vi "Sort 2D String Array - Sort Data.vi"(0 "Array to sort in":string[][](array[string]), 3 "Column Sort Order":i32[](array[numeric]), 4 "Input Array Contains Header Row? (T)":T1) -> (14 "Sorted Array (Cols in Original Order. Header row removed)":T2, 15 "Sorted Array (Cols in Sort Order. Header row removed)":T4, 16 "Sorted Array (Cols in Sort Order. Headers as last row)":T3)   [LabVIEW 2009, in "xijk_select_best_filter.lvlib"]
doc: "Sort 2D String Array - Sort Data.vi\n\n<B>Description:</B>\n\nThis VI sorts an array of strings in the order specified by the Column Sort Order input.\n\n<B>Usage:</B>\n\nWire all required inputs.\n\n<B>Inputs:</B>\n\nArray to Sort In\n- This is the input array of strings that will be sorted.\n\nColumn Sort Order\n- This control specifies the column sort order. If it is left unwired, the sort order will be 0,1,2...\n\nInput Array Contains Header Row? (T)\n- This input indicates if the input array contains a header row.\n\n<B>Outputs:</B>\n\nSorted Array (Cols in Original Order. Header row removed)\n- This is the input array of strings sorted in the order specified by the Column Sort Order input with the columns in the original order and the header row removed.\n\nSorted Array (Cols in Sort Order. Header row removed)\n- This is the input array of strings sorted in the order specified by the Column Sort Order input with the columns in the order specified by the Column Sort Order input and the header row removed.\n\nSorted Array (Cols in Sort Order. Headers as last row)\n- This is the input array of strings sorted in the order specified by the Column Sort Order input with the columns in the order specified by the Column Sort Order input and the header row positioned as the last row of the array.\n\n<B>Developed by:</B>\n\nMark Ridgley\nmark.ridgley@logicpd.com"
uses:
  xijk_select_best_filter.lvlib
  _TypeDefs/TYPE - Sorted Array (Cols in Original Order. Header row removed).ctl
  _TypeDefs/TYPE - Sorted Array (Cols in Sort Order. Header row removed).ctl
  _TypeDefs/TYPE - Sorted Array (Cols in Sort Order. Headers as last row).ctl
  _TypeDefs/TYPE - Input Array Contains Header Row.ctl
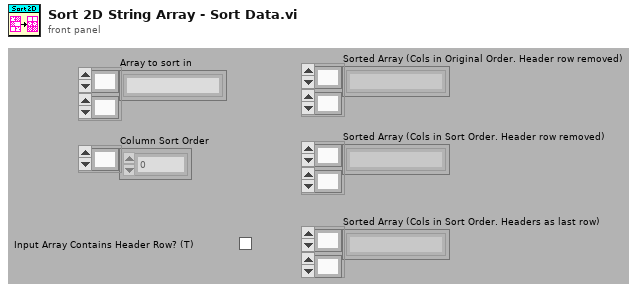
[diagram p1: front panel]
types:
  T1 = typedef "xijk_select_best_filter.lvlib/TYPE - Input Array Contains Header Row.ctl" = bool
  T2 = typedef "xijk_select_best_filter.lvlib/TYPE - Sorted Array (Cols in Original Order. Header row removed).ctl" = string[][]
  T3 = typedef "xijk_select_best_filter.lvlib/TYPE - Sorted Array (Cols in Sort Order. Headers as last row).ctl" = string[][]
  T4 = typedef "xijk_select_best_filter.lvlib/TYPE - Sorted Array (Cols in Sort Order. Header row removed).ctl" = string[][]
  T5 = cluster{"Output String (\" \")":string, "Output String (\" \")":string, "Output String (\" \")":string, "Output String (\" \")":string, "Output String (\" \")":string, "Output String (\" \")":string, "Output String (\" \")":string, "Output String (\" \")":string, "Output String (\" \")":string, "Output String (\" \")":string, "Output String (\" \")":string, "Output String (\" \")":string, "Output String (\" \")":string, "Output String (\" \")":string, "Output String (\" \")":string, "Output String (\" \")":string, "Output String (\" \")":string, "Output String (\" \")":string, "Output String (\" \")":string, "Output String (\" \")":string, "Output String (\" \")":string, "Output String (\" \")":string, "Output String (\" \")":string, "Output String (\" \")":string, "Output String (\" \")":string, "Output String (\" \")":string, "Output String (\" \")":string, "Output String (\" \")":string, "Output String (\" \")":string, "Output String (\" \")":string, "Output String (\" \")":string, "Output String (\" \")":string, "Output String (\" \")":string, "Output String (\" \")":string, "Output String (\" \")":string, "Output String (\" \")":string, "Output String (\" \")":string, "Output String (\" \")":string, "Output String (\" \")":string, "Output String (\" \")":string, "Output String (\" \")":string, "Output String (\" \")":string, "Output String (\" \")":string, "Output String (\" \")":string, "Output String (\" \")":string, "Output String (\" \")":string, "Output String (\" \")":string, "Output String (\" \")":string, "Output String (\" \")":string, "Output String (\" \")":string, "Output String (\" \")":string, "Output String (\" \")":string, "Output String (\" \")":string, "Output String (\" \")":string, "Output String (\" \")":string, "Output String (\" \")":string, "Output String (\" \")":string, "Output String (\" \")":string, "Output String (\" \")":string, "Output String (\" \")":string, "Output String (\" \")":string, "Output String (\" \")":string, "Output String (\" \")":string, "Output String (\" \")":string, "Output String (\" \")":string, "Output String (\" \")":string, "Output String (\" \")":string, "Output String (\" \")":string, "Output String (\" \")":string, "Output String (\" \")":string, "Output String (\" \")":string, "Output String (\" \")":string, "Output String (\" \")":string, "Output String (\" \")":string, "Output String (\" \")":string, "Output String (\" \")":string, "Output String (\" \")":string, "Output String (\" \")":string, "Output String (\" \")":string, "Output String (\" \")":string, "Output String (\" \")":string, "Output String (\" \")":string, "Output String (\" \")":string, "Output String (\" \")":string, "Output String (\" \")":string, "Output String (\" \")":string, "Output String (\" \")":string, "Output String (\" \")":string, "Output String (\" \")":string, "Output String (\" \")":string, "Output String (\" \")":string, "Output String (\" \")":string, "Output String (\" \")":string, "Output String (\" \")":string, "Output String (\" \")":string, "Output String (\" \")":string, "Output String (\" \")":string, "Output String (\" \")":string, "Output String (\" \")":string, "Output String (\" \")":string, "Output String (\" \")":string, "Output String (\" \")":string, "Output String (\" \")":string, "Output String (\" \")":string, "Output String (\" \")":string, "Output String (\" \")":string, "Output String (\" \")":string, "Output String (\" \")":string, "Output String (\" \")":string, "Output String (\" \")":string, "Output String (\" \")":string, "Output String (\" \")":string, "Output String (\" \")":string, "Output String (\" \")":string, "Output String (\" \")":string, "Output String (\" \")":string, "Output String (\" \")":string, "Output String (\" \")":string, "Output String (\" \")":string, "Output String (\" \")":string, "Output String (\" \")":string, "Output String (\" \")":string, "Output String (\" \")":string, "Output String (\" \")":string, "Output String (\" \")":string, "Output String (\" \")":string, "Output String (\" \")":string, "Output String (\" \")":string, "Output String (\" \")":string, "Output String (\" \")":string, "Output String (\" \")":string, "Output String (\" \")":string, "Output String (\" \")":string, "Output String (\" \")":string, "Output String (\" \")":string, "Output String (\" \")":string, "Output String (\" \")":string, "Output String (\" \")":string, "Output String (\" \")":string, "Output String (\" \")":string, "Output String (\" \")":string, "Output String (\" \")":string, "Output String (\" \")":string, "Output String (\" \")":string, "Output String (\" \")":string, "Output String (\" \")":string, "Output String (\" \")":string, "Output String (\" \")":string, "Output String (\" \")":string, "Output String (\" \")":string, "Output String (\" \")":string, "Output String (\" \")":string, "Output String (\" \")":string, "Output String (\" \")":string, "Output String (\" \")":string, "Output String (\" \")":string, "Output String (\" \")":string, "Output String (\" \")":string, "Output String (\" \")":string, "Output String (\" \")":string, "Output String (\" \")":string, "Output String (\" \")":string, "Output String (\" \")":string, "Output String (\" \")":string, "Output String (\" \")":string, "Output String (\" \")":string, "Output String (\" \")":string, "Output String (\" \")":string, "Output String (\" \")":string, "Output String (\" \")":string, "Output String (\" \")":string, "Output String (\" \")":string, "Output String (\" \")":string, "Output String (\" \")":string, "Output String (\" \")":string, "Output String (\" \")":string, "Output String (\" \")":string, "Output String (\" \")":string, "Output String (\" \")":string, "Output String (\" \")":string, "Output String (\" \")":string, "Output String (\" \")":string, "Output String (\" \")":string, "Output String (\" \")":string, "Output String (\" \")":string, "Output String (\" \")":string, "Output String (\" \")":string, "Output String (\" \")":string, "Output String (\" \")":string, "Output String (\" \")":string, "Output String (\" \")":string, "Output String (\" \")":string, "Output String (\" \")":string, "Output String (\" \")":string, "Output String (\" \")":string, "Output String (\" \")":string, "Output String (\" \")":string, "Output String (\" \")":string, "Output String (\" \")":string, "Output String (\" \")":string, "Output String (\" \")":string, "Output String (\" \")":string, "Output String (\" \")":string, "Output String (\" \")":string, "Output String (\" \")":string, "Output String (\" \")":string, "Output String (\" \")":string, "Output String (\" \")":string, "Output String (\" \")":string, "Output String (\" \")":string, "Output String (\" \")":string, "Output String (\" \")":string, "Output String (\" \")":string, "Output String (\" \")":string, "Output String (\" \")":string, "Output String (\" \")":string, "Output String (\" \")":string, "Output String (\" \")":string, "Output String (\" \")":string, "Output String (\" \")":string, "Output String (\" \")":string, "Output String (\" \")":string, "Output String (\" \")":string, "Output String (\" \")":string, "Output String (\" \")":string, "Output String (\" \")":string, "Output String (\" \")":string, "Output String (\" \")":string, "Output String (\" \")":string, "Output String (\" \")":string, "Output String (\" \")":string, "Output String (\" \")":string, "Output String (\" \")":string, "Output String (\" \")":string, "Output String (\" \")":string, "Output String (\" \")":string, "Output String (\" \")":string, "Output String (\" \")":string, "Output String (\" \")":string, "Output String (\" \")":string, "Output String (\" \")":string, "Output String (\" \")":string, "Output String (\" \")":string, "Output String (\" \")":string, "Output String (\" \")":string, "Output String (\" \")":string, "Output String (\" \")":string, "Output String (\" \")":string, "Output String (\" \")":string, "Output String (\" \")":string, "Output String (\" \")":string, "Output String (\" \")":string, "Output String (\" \")":string, "Output String (\" \")":string, "Output String (\" \")":string, "Output String (\" \")":string}[]
  T6 = cluster{"[0]":string, "[1]":string, "[2]":string, "[3]":string, "[4]":string, "[5]":string, "[6]":string, "[7]":string, "[8]":string, "[9]":string, "[10]":string, "[11]":string, "[12]":string, "[13]":string, "[14]":string, "[15]":string, "[16]":string, "[17]":string, "[18]":string, "[19]":string, "[20]":string, "[21]":string, "[22]":string, "[23]":string, "[24]":string, "[25]":string, "[26]":string, "[27]":string, "[28]":string, "[29]":string, "[30]":string, "[31]":string, "[32]":string, "[33]":string, "[34]":string, "[35]":string, "[36]":string, "[37]":string, "[38]":string, "[39]":string, "[40]":string, "[41]":string, "[42]":string, "[43]":string, "[44]":string, "[45]":string, "[46]":string, "[47]":string, "[48]":string, "[49]":string, "[50]":string, "[51]":string, "[52]":string, "[53]":string, "[54]":string, "[55]":string, "[56]":string, "[57]":string, "[58]":string, "[59]":string, "[60]":string, "[61]":string, "[62]":string, "[63]":string, "[64]":string, "[65]":string, "[66]":string, "[67]":string, "[68]":string, "[69]":string, "[70]":string, "[71]":string, "[72]":string, "[73]":string, "[74]":string, "[75]":string, "[76]":string, "[77]":string, "[78]":string, "[79]":string, "[80]":string, "[81]":string, "[82]":string, "[83]":string, "[84]":string, "[85]":string, "[86]":string, "[87]":string, "[88]":string, "[89]":string, "[90]":string, "[91]":string, "[92]":string, "[93]":string, "[94]":string, "[95]":string, "[96]":string, "[97]":string, "[98]":string, "[99]":string, "[100]":string, "[101]":string, "[102]":string, "[103]":string, "[104]":string, "[105]":string, "[106]":string, "[107]":string, "[108]":string, "[109]":string, "[110]":string, "[111]":string, "[112]":string, "[113]":string, "[114]":string, "[115]":string, "[116]":string, "[117]":string, "[118]":string, "[119]":string, "[120]":string, "[121]":string, "[122]":string, "[123]":string, "[124]":string, "[125]":string, "[126]":string, "[127]":string, "[128]":string, "[129]":string, "[130]":string, "[131]":string, "[132]":string, "[133]":string, "[134]":string, "[135]":string, "[136]":string, "[137]":string, "[138]":string, "[139]":string, "[140]":string, "[141]":string, "[142]":string, "[143]":string, "[144]":string, "[145]":string, "[146]":string, "[147]":string, "[148]":string, "[149]":string, "[150]":string, "[151]":string, "[152]":string, "[153]":string, "[154]":string, "[155]":string, "[156]":string, "[157]":string, "[158]":string, "[159]":string, "[160]":string, "[161]":string, "[162]":string, "[163]":string, "[164]":string, "[165]":string, "[166]":string, "[167]":string, "[168]":string, "[169]":string, "[170]":string, "[171]":string, "[172]":string, "[173]":string, "[174]":string, "[175]":string, "[176]":string, "[177]":string, "[178]":string, "[179]":string, "[180]":string, "[181]":string, "[182]":string, "[183]":string, "[184]":string, "[185]":string, "[186]":string, "[187]":string, "[188]":string, "[189]":string, "[190]":string, "[191]":string, "[192]":string, "[193]":string, "[194]":string, "[195]":string, "[196]":string, "[197]":string, "[198]":string, "[199]":string, "[200]":string, "[201]":string, "[202]":string, "[203]":string, "[204]":string, "[205]":string, "[206]":string, "[207]":string, "[208]":string, "[209]":string, "[210]":string, "[211]":string, "[212]":string, "[213]":string, "[214]":string, "[215]":string, "[216]":string, "[217]":string, "[218]":string, "[219]":string, "[220]":string, "[221]":string, "[222]":string, "[223]":string, "[224]":string, "[225]":string, "[226]":string, "[227]":string, "[228]":string, "[229]":string, "[230]":string, "[231]":string, "[232]":string, "[233]":string, "[234]":string, "[235]":string, "[236]":string, "[237]":string, "[238]":string, "[239]":string, "[240]":string, "[241]":string, "[242]":string, "[243]":string, "[244]":string, "[245]":string, "[246]":string, "[247]":string, "[248]":string, "[249]":string, "[250]":string, "[251]":string, "[252]":string, "[253]":string, "[254]":string, "[255]":string}
  T7 = cluster{"[0]":string, "[1]":string, "[2]":string, "[3]":string, "[4]":string, "[5]":string, "[6]":string, "[7]":string, "[8]":string, "[9]":string, "[10]":string, "[11]":string, "[12]":string, "[13]":string, "[14]":string, "[15]":string, "[16]":string, "[17]":string, "[18]":string, "[19]":string, "[20]":string, "[21]":string, "[22]":string, "[23]":string, "[24]":string, "[25]":string, "[26]":string, "[27]":string, "[28]":string, "[29]":string, "[30]":string, "[31]":string, "[32]":string, "[33]":string, "[34]":string, "[35]":string, "[36]":string, "[37]":string, "[38]":string, "[39]":string, "[40]":string, "[41]":string, "[42]":string, "[43]":string, "[44]":string, "[45]":string, "[46]":string, "[47]":string, "[48]":string, "[49]":string, "[50]":string, "[51]":string, "[52]":string, "[53]":string, "[54]":string, "[55]":string, "[56]":string, "[57]":string, "[58]":string, "[59]":string, "[60]":string, "[61]":string, "[62]":string, "[63]":string, "[64]":string, "[65]":string, "[66]":string, "[67]":string, "[68]":string, "[69]":string, "[70]":string, "[71]":string, "[72]":string, "[73]":string, "[74]":string, "[75]":string, "[76]":string, "[77]":string, "[78]":string, "[79]":string, "[80]":string, "[81]":string, "[82]":string, "[83]":string, "[84]":string, "[85]":string, "[86]":string, "[87]":string, "[88]":string, "[89]":string, "[90]":string, "[91]":string, "[92]":string, "[93]":string, "[94]":string, "[95]":string, "[96]":string, "[97]":string, "[98]":string, "[99]":string, "[100]":string, "[101]":string, "[102]":string, "[103]":string, "[104]":string, "[105]":string, "[106]":string, "[107]":string, "[108]":string, "[109]":string, "[110]":string, "[111]":string, "[112]":string, "[113]":string, "[114]":string, "[115]":string, "[116]":string, "[117]":string, "[118]":string, "[119]":string, "[120]":string, "[121]":string, "[122]":string, "[123]":string, "[124]":string, "[125]":string, "[126]":string, "[127]":string, "[128]":string, "[129]":string, "[130]":string, "[131]":string, "[132]":string, "[133]":string, "[134]":string, "[135]":string, "[136]":string, "[137]":string, "[138]":string, "[139]":string, "[140]":string, "[141]":string, "[142]":string, "[143]":string, "[144]":string, "[145]":string, "[146]":string, "[147]":string, "[148]":string, "[149]":string, "[150]":string, "[151]":string, "[152]":string, "[153]":string, "[154]":string, "[155]":string, "[156]":string, "[157]":string, "[158]":string, "[159]":string, "[160]":string, "[161]":string, "[162]":string, "[163]":string, "[164]":string, "[165]":string, "[166]":string, "[167]":string, "[168]":string, "[169]":string, "[170]":string, "[171]":string, "[172]":string, "[173]":string, "[174]":string, "[175]":string, "[176]":string, "[177]":string, "[178]":string, "[179]":string, "[180]":string, "[181]":string, "[182]":string, "[183]":string, "[184]":string, "[185]":string, "[186]":string, "[187]":string, "[188]":string, "[189]":string, "[190]":string, "[191]":string, "[192]":string, "[193]":string, "[194]":string, "[195]":string, "[196]":string, "[197]":string, "[198]":string, "[199]":string, "[200]":string, "[201]":string, "[202]":string, "[203]":string, "[204]":string, "[205]":string, "[206]":string, "[207]":string, "[208]":string, "[209]":string, "[210]":string, "[211]":string, "[212]":string, "[213]":string, "[214]":string, "[215]":string, "[216]":string, "[217]":string, "[218]":string, "[219]":string, "[220]":string, "[221]":string, "[222]":string, "[223]":string, "[224]":string, "[225]":string, "[226]":string, "[227]":string, "[228]":string, "[229]":string, "[230]":string, "[231]":string, "[232]":string, "[233]":string, "[234]":string, "[235]":string, "[236]":string, "[237]":string, "[238]":string, "[239]":string, "[240]":string, "[241]":string, "[242]":string, "[243]":string, "[244]":string, "[245]":string, "[246]":string, "[247]":string, "[248]":string, "[249]":string, "[250]":string, "[251]":string, "[252]":string, "[253]":string, "[254]":string, "[255]":string}[]
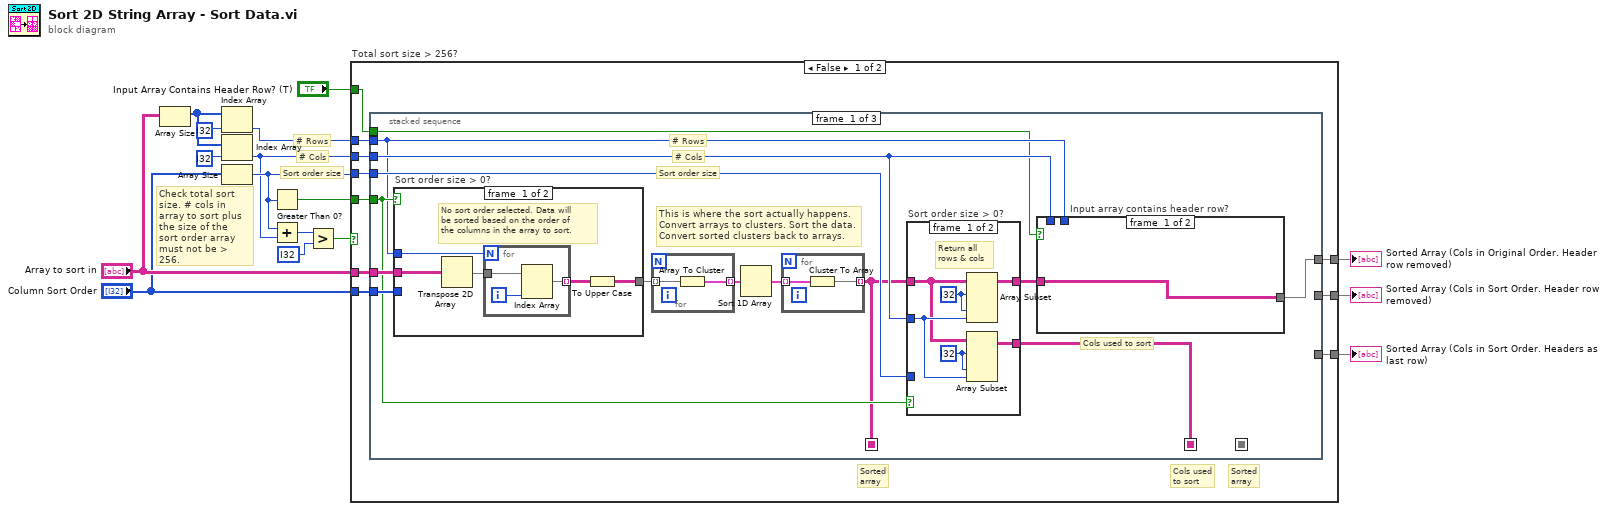
[diagram p0: block diagram]
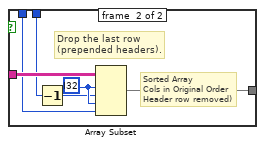
[diagram p2: hidden frame]
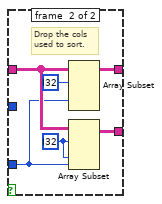
[diagram p3: hidden frame]
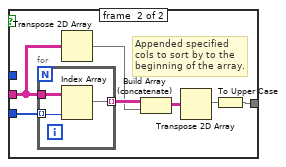
[diagram p4: hidden frame]
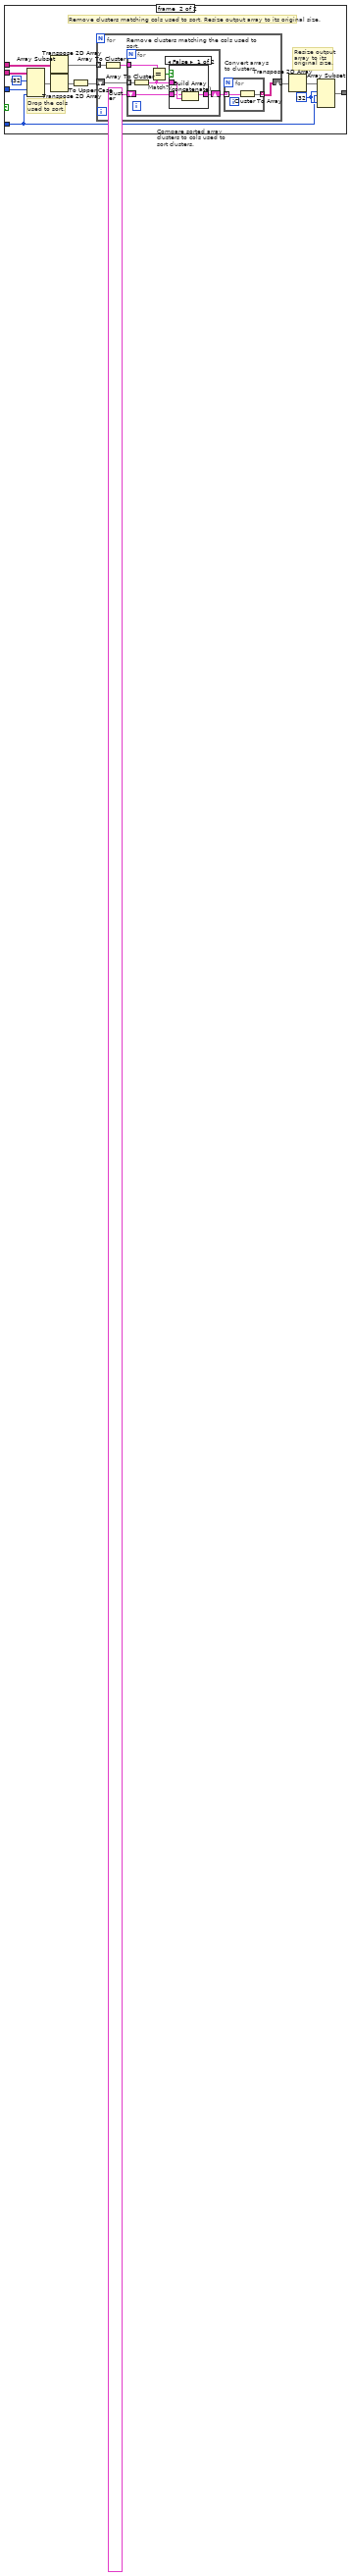
[diagram p6: hidden frame]
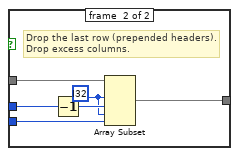
[diagram p9: hidden frame]
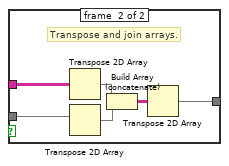
[diagram p10: hidden frame]
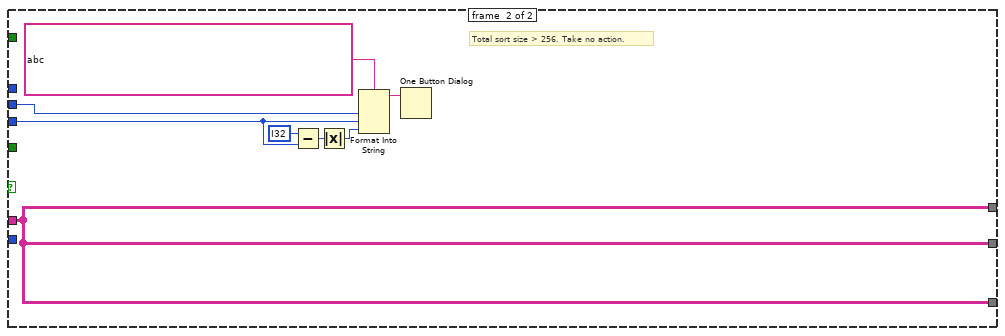
[diagram p11: hidden frame]
diagram:
  # "Check total sort\nsize. # cols in\narray to sort plus\nthe size of the\nsort order array\nmust not be > 256."
  # "# Rows"
  # "# Cols"
  # "Sort order size"
  n1 = Array Size(array="Array to sort in") -> (size(s)=w11:i32[])
  n2 = Index Array(array=w11, index=i32 ?) -> (element=w8:i32)
  n3 = Index Array(array=w11, index=i32 ?) -> (element=w2:i32)
  n4 = Array Size(array="Column Sort Order") -> (size(s)=w4:i32)
  n5 = Greater Than 0?(x=w4) -> (x > 0?=w3:bool)
  n6 = Add(x=w4, y=w2) -> (x+y=w10:i32)
  n7 = Greater?(x=w10, y=i32 ?) -> (0:w5:bool)
  n8 = case "Total sort size > 256?" shown="False" w5 {
    tunnel: [w26 w149] -> w16
    tunnel: [w25 w149] -> w15
    tunnel: [w24 w149] -> w14
    tunnel: w8 -> [w23 _]
    tunnel: w2 -> [w22 w142]
    tunnel: w4 -> [w21 w143]
    tunnel: "Array to sort in" -> [w20 w149]
    tunnel: "Column Sort Order" -> [w19 _]
    tunnel: w3 -> [w18 _]
    tunnel: "Input Array Contains Header Row? (T)" -> [w17 _]
    frame #0 {
      # "Sorted\narray"
      # "Cols used\nto sort"
      # "Sorted\narray"
      n9 = stacked-sequence {
        seq-local: [w27 _ _] -> [_ w84 _]
        seq-local: [w33 _ _] -> [_ w82 w126]
        seq-local: [_ w83 _] -> [_ _ w127]
        tunnel: w23 -> [w30 w86 w123]
        tunnel: w20 -> [w40 _ _]
        tunnel: w19 -> [w39 _ _]
        tunnel: w18 -> [w34 w87 w121]
        tunnel: w21 -> [w32 w85 _]
        tunnel: [w29 _ _] -> w24
        tunnel: w22 -> [w31 _ w122]
        tunnel: [_ _ w124] -> w25
        tunnel: [_ _ w125] -> w26
        tunnel: w17 -> [w28 _ w120]
        frame #0 {
          # "Cols used to sort"
          # "# Rows"
          # "# Cols"
          # "Sort order size"
          # "This is where the sort actually happens.\nConvert arrays to clusters. Sort the data.\nConvert sorted clusters back to arrays."
          n10 = case "Sort order size > 0?" shown="True" w34 {
            tunnel: w40 -> [w68 w78]
            tunnel: [w64 w72] -> w36
            tunnel: w39 -> [_ w75]
            tunnel: w30 -> [w67 _]
            frame #0 {
              # "No sort order selected. Data will\nbe sorted based on the order of\nthe columns in the array to sort."
              n11 = Transpose 2D Array(2D array=w68) -> (transposed array=w66:string[][])
              n12 = for {
                N: w67 -> [_]
                tunnel: w66 -> [w71]
                tunnel: [w69] -> w65 mode=indexing
                i -> [w70]
                n13 = Index Array(array=w71, index (col)=w70) -> (element=w69:string[])  [unwired: 1 in]
              }
              n14 = To Upper Case(1:w65) -> (0:w64:string[][])
            }
            frame #1 {
              # "Appended specified\ncols to sort by to the\nbeginning of the array."
              n15 = for {
                tunnel: w78 -> [w81]
                tunnel: [w79] -> w77 mode=indexing
                tunnel: w75 -> [w80] mode=indexing
                n16 = Index Array(array=w81, index (col)=w80) -> (element=w79:string[])  [unwired: 1 in]
              }
              n17 = Transpose 2D Array(2D array=w78) -> (transposed array=w76:string[][])
              n18 = Build Array (concatenate)(w77, w76) -> (w74:string[][])
              n19 = Transpose 2D Array(2D array=w74) -> (transposed array=w73:string[][])
              n20 = To Upper Case(1:w73) -> (0:w72:string[][])
            }
          }
          n21 = for {
            tunnel: w36 -> [w62] mode=indexing
            tunnel: [w63] -> w37 mode=indexing
            n22 = Array To Cluster(array=w62) -> (cluster=w63:T6)
          }
          n23 = Sort 1D Array(array=w37) -> (sorted array=w38:T7)
          n24 = for {
            tunnel: w38 -> [w61] mode=indexing
            tunnel: [w60] -> w27 mode=indexing
            n25 = Cluster To Array(cluster=w61) -> (array=w60:string[])
          }
          n26 = case "Sort order size > 0?" shown="True" w34 {
            tunnel: w27 -> [w48 w56]
            tunnel: [w53 w58] -> w35
            tunnel: w32 -> [_ w55]
            tunnel: w31 -> [w49 _]
            tunnel: [w50 w54] -> w33
            frame #0 {
              w51 = i32 ? ("Array Index")
              w52 = i32 ? ("Array Index")
              # "Return all\nrows & cols"
              n27 = Array Subset(array=w48, index (row)=w52, index (col)=w52, length (col)=w49) -> (w53:string[][])  [unwired: 1 in]
              n28 = Array Subset(array=w48, index (row)=w51, index (col)=w51, length (col)=w49) -> (w50:string[][])  [unwired: 1 in]
            }
            frame #1 {
              w57 = i32 ? ("Array Index")
              # "Drop the cols\nused to sort."
              n29 = Array Subset(array=w56, index (row)=i32 ? ("Array Index"), index (col)=w55) -> (w58:string[][])  [unwired: 2 in]
              n30 = Array Subset(array=w56, index (row)=w57, index (col)=w57, length (col)=w55) -> (w54:string[][])  [unwired: 1 in]
            }
          }
          n31 = case "Input array contains header row?" shown="True" w28 {
            tunnel: w35 -> [w41 w45]
            tunnel: w31 -> [_ w44]
            tunnel: w30 -> [_ w43]
            tunnel: [w41 w42] -> w29
            frame #0 {
            }
            frame #1 {
              w47 = i32 ? ("Array Index")
              # "Sorted Array\nCols in Original Order\nHeader row removed)"
              # "Drop the last row\n(prepended headers)."
              n32 = Decrement(x=w43) -> (x-1=w46:i32)
              n33 = Array Subset(array=w45, index (row)=w47, length (row)=w46, index (col)=w47, length (col)=w44) -> (w42:string[][])
            }
          }
        }
        frame #1 {
          # "Sort order size > 0?"
          # "Sort order size"
          # "# Rows"
          # "Sorted array"
          # "Cols used to sort"
          n34 = case "Sort order size > 0?" shown="True" w87 {
            tunnel: [w88 w99] -> w83
            tunnel: w82 -> [w88 w89]
            tunnel: w86 -> [_ w92]
            tunnel: w84 -> [_ w93]
            tunnel: w85 -> [_ w91]
            frame #0 {
              # "Sort order size is not > 0.\nCols used to sort is the sorted array.\nPass it to the output."
            }
            frame #1 {
              w101 = i32 ? ("Array Index")
              # "Remove clusters matching cols used to sort. Resize output array to its original size."
              # "Resize output\narray to its\noriginal size."
              # "Drop the cols\nused to sort."
              n35 = Array Subset(array=w93, index (row)=i32 ? ("Array Index"), index (col)=w91, length (col)=w92) -> (w96:string[][])  [unwired: 1 in]
              n36 = Transpose 2D Array(2D array=w89) -> (transposed array=w90:string[][])
              n37 = Transpose 2D Array(2D array=w96) -> (transposed array=w97:string[][])
              n38 = To Upper Case(1:w97) -> (0:w94:string[][])
              n39 = for "Compare sorted array clusters to cols used to sort clusters." {
                tunnel: w90 -> [w106] mode=indexing
                shift-right: [w103] -> w98
                shift-left: w94 -> [w102]
                n40 = Array To Cluster(array=w106) -> (cluster=w105:T6)
                n41 = for "Remove clusters matching the cols used to sort." {
                  tunnel: w102 -> [w115] mode=indexing
                  tunnel: w105 -> [w111]
                  shift-right: [w112] -> w104
                  shift-left: T5 ? -> [w113]
                  n42 = Array To Cluster(array=w115) -> (cluster=w110:T6)
                  n43 = Equal?(x=w111, y=w110) -> (x = y?=w114:bool)
                  n44 = case "Match?" shown="False" w114 {
                    tunnel: w110 -> [w118 _]
                    tunnel: [w117 w119] -> w112
                    tunnel: w113 -> [w116 w119]
                    frame #0 {
                      n45 = Build Array (concatenate)(w116, w118) -> (w117:T7)
                    }
                    frame #1 {
                    }
                  }
                }
                n46 = for "Convert arrays\nto clusters." {
                  tunnel: w104 -> [w109] mode=indexing
                  tunnel: [w108] -> w103 mode=indexing
                  n47 = Cluster To Array(cluster=w109) -> (array=w108:string[])
                }
              }
              n48 = Transpose 2D Array(2D array=w98) -> (transposed array=w100:string[][])
              n49 = Array Subset(array=w100, index (row)=w101, length (row)=w92, index (col)=w101) -> (w99:string[][])  [unwired: 1 in]
            }
          }
        }
        frame #2 {
          # "Sorted Array (Cols in Sort Order. Headers as last row)"
          # "Sorted Array (Cols in Sort Order)"
          # "Sorted array"
          # "Cols used to sort"
          # "Sort order size > 0?"
          # "# Cols"
          # "# Rows"
          n50 = case "Sort order size > 0?" shown="True" w121 {
            tunnel: w126 -> [w135 w139]
            tunnel: w127 -> [_ w138]
            tunnel: [w135 w136] -> w124
            frame #0 {
              # "Sort order size is not > 0.\nCols used to sort is the sorted array.\nPass it to the output."
            }
            frame #1 {
              # "Transpose and join arrays."
              n51 = Transpose 2D Array(2D array=w139) -> (transposed array=w140:string[][])
              n52 = Transpose 2D Array(2D array=w138) -> (transposed array=w137:string[][])
              n53 = Build Array (concatenate)(w140, w137) -> (w141:string[][])
              n54 = Transpose 2D Array(2D array=w141) -> (transposed array=w136:string[][])
            }
          }
          n55 = case "Input array contains header row?" shown="True" w120 {
            tunnel: w123 -> [_ w132]
            tunnel: w122 -> [_ w131]
            tunnel: [w128 w130] -> w125
            tunnel: w124 -> [w128 w129]
            frame #0 {
              # "No header rows to remove.\nPass array to output."
            }
            frame #1 {
              w133 = i32 ? ("Array Index")
              # "Drop the last row (prepended headers).\nDrop excess columns."
              n56 = Decrement(x=w132) -> (x-1=w134:i32)
              n57 = Array Subset(array=w129, index (row)=w133, length (row)=w134, index (col)=w133, length (col)=w131) -> (w130:string[][])
            }
          }
        }
      }
    }
    frame #1 {
      # "Total sort size > 256. Take no action."
      n58 = Subtract(x=i32 ?, y=w143) -> (x-y=w146:i32)
      n59 = Absolute Value(x=w146) -> (abs(x)=w145:i32)
      n60 = Format Into String(format string=string ? ("message"), w142, w143, w145) -> (resulting string=w148:string)  [unwired: 2 in, 1 out]
      n61 = One Button Dialog(message=w148) -> ()  [unwired: 2 out]
    }
  }
  "Sorted Array (Cols in Sort Order. Header row removed)" <- w16
  "Sorted Array (Cols in Sort Order. Headers as last row)" <- w15
  "Sorted Array (Cols in Original Order. Header row removed)" <- w14
